vi "NIMS_NS_fir_minphase.vi"(5 "Function name":string, 6 "Line number":i32, 7 "Number of outputs requested":i32, 8 "error in (no error)":errorcluster, 11 "[A]":variant[](array[variant])) -> (0 "error out":errorcluster, 3 "[funct(A)]":variant[](array[variant]))   [LabVIEW 2017]
uses:
  <vilib>/imath/engines/lvmath/Functions/Error Handling/error.ctl
  <instcachedir>/0/NIMS_RunTimeType_From StrictType (excl LVString)_1019F277F0A747EDBCA0F6C52CA54500.lvgen/NIMS_RunTimeType_From StrictType (excl LVString)_1019F277F0A747EDBCA0F6C52CA54500_000.vi
  <instcachedir>/0/NIMS_Get Any Vector_w Error - Matrix_9FDB8FBE264C42EDBC8FF9BA66C3EF33.lvgen/NIMS_Get Any Vector_w Error - Matrix_9FDB8FBE264C42EDBC8FF9BA66C3EF33_001.vi
  <instcachedir>/0/NIMS_Complex To Real_BE01396FDE034E8E94CEBBA1E368668D.lvgen/NIMS_Complex To Real_BE01396FDE034E8E94CEBBA1E368668D_000.vi
  <instcachedir>/0/NIMS_RunTimeType_To Numeric_1CBDAFC4EFAD4045A1DE52278D16738D.lvgen/NIMS_RunTimeType_To Numeric_1CBDAFC4EFAD4045A1DE52278D16738D_000.vi
  <vilib>/addons/Digital Filter Design/NI_DigFilter_MathScript.lvlib
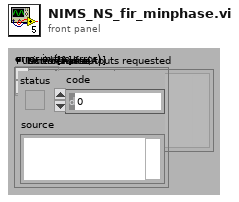
[diagram p1: front panel]
types:
  T1 = typedef "error.ctl" = enum16{"No Error", "Problem", "Input type must not be void", "Incorrect number of parameters", "Function not defined for non-numeric types", "An output variable of the user-defined function is undefined", "Function only defined for character arrays", "Function not defined for boolean, character, or single precision", "Function not defined for complex types", "Not a valid operation", "Inputs must be scalar", "Input matrices are not the same size", "Function only available on RT", "Input matrices must be nonnegative integers of the same type", "Arguments must be non-negative integers less than bitmax", "Number to complement must be less than 2^N", "Bit to get is outside range", "Bit to set is outside range", "Input must be real type ", "At least one parameter must be scalar", "Unable to display plug-in data on RT", "Function not defined for higher dimensional matrices", "Invalid attributes", "Wrong Type of Input Arguments", "Wrong Argument Option", "Invalid file identifier", "Indices must be real positive integers", "The variable is not a matrix data type.", "Number of elements must be the same for indices and values", "You cannot replace elements of a matrix with non-matrix data types.", "Cannot resize a 2D matrix with a linear index", "Unknown variable or symbol", "Indices out of range", "Empty matrix deletion can not be used with two indices", "Number of rows and columns must be the same for indices and values.", "Complex cannot be converted to Boolean", "Char cannot be converted to Boolean", "int64 cannot be converted to Boolean", "uint64 cannot be converted to Boolean", "You cannot convert a Boolean to a character.", "Incompatible input size in 3D surface function", "All rows must have the same number of columns", "Incompatible types", "Invalid matrix dimensions", "Dimension must be 1 or 2", "Base must be an integer between 2 and 36", "Invalid input", "Square matrix required", "Function 'timerstart' must be called before 'timerstop'", "Arguments must be positive real", "Step must not be zero", "Wrong number of input arguments", "Wrong number of output arguments", "Too many index arguments", "Input scalar must be >= 0", "Input scalar must be positive", "Input scalar must not be 0", "Input scalar must be in range [0,1]", "Can't use conditionally defined variable that's undefined", "Input must be a vector", "RT Exec Trace Toolkit not licensed", "Empty vector error", "All elements must be in domain [-1,1]", "All real elements of input vector must be >= 0", "All elements of input vector must be positive", "Values of input vectors are not compatible", "DAQmx not installed", "Input vector must be an increasing vector", "Dereferenced field does not exist within the struct", "A vector or matrix of structures must be indexed before it can be dereferenced", "Lenths of two input vectors are not compatible", "Invalid fieldname", "Empty matrix error", "Cannot use '.' on a type other than Struct", "Unused074", "Data type of the struct's field name is invalid", "Using . to dereference data that is not a struct", "Input struct contains invalid type ", "Size of input matrix is incompatible with input size", "Invalid format specifier", "Could not find field within struct", "Bad permutation array", "Mismatched fieldnames", "ode: User Function could not be opened", "ode: User Function signature does not meet ode requirements", "Unused085", "RunTime: MathScript could not be compiled", "Unknown function", "Only scalars and strings supported", "ode: User Function signature has incorrect number of inputs", "ode:User Function signature has incorrect number of outputs", "Range is too large", "End used without variable", "Function not available (RTE)", "Custom user error", "Arguments must be integers less than bitmax", "Shared library not found", "Header file not found", "Shared library already loaded", "Shared library not loaded", "Shared library function not found", "Shared library string return problem", "Problem calling shared library function", "Problem loading shared library from OS", "Problem parsing shared library header file", "Shared library incompatible types", "Shared library unsupported return type", "Shared library function not exported", "Shared library unsupported input type", "Problem unloading shared library from OS", "Function only available from UI", "Function specified in argument is missing", "An internal error has occurred", "Invalid object", "Invalid property", "Read-only property", "A break command has occurred", "A continue command has occurred", "A return command has occurred", "ode: times parameter invalid", "Function specified in argument has incorrect signature", "Function not found in file", "Reserved keyword cannot be defined as variable", "Reserved keyword cannot be defined as a function or script", "Arguments must be string literals", "Function not supported on this platform", "All columns must have the same number of rows", "Function ignored in RTE warning", "Cannot use : as a parameter that is not a variable", "Output can't be coerced to requested type", "Function not supported on current target", "Variable dependent on an unwired function input", "Unused132", "Unused133", "Unused134", "Unused135", "Unused136", "Unused137", "Unused138", "Unused139", "Global/Persistent must only take constants as arguments.", "Varargin must be last input in the function definition.", "Varargout must be last output in the function definition.", "Invalid output type. Cannot output a cell array of any type other than string.", "Invalid output type. Type is a dynamic struct.", "Invalid output type. Type is a struct that has a field whose type is not known until run-time", "Invalid output type. Type is a struct that has a field which is a plot object.", "MathScript parser DLL missing", "MathScript requires LabVIEW Full", "MathScript license is invalid or missing", "Varargout not supported except in assignments."}
  T2 = typedef "NIMS_CH_character datatype.ctl" = cluster{"Numeric":u8}
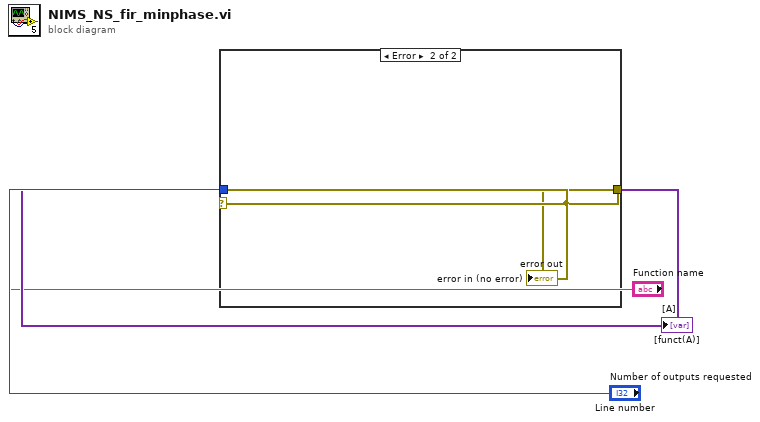
[diagram p0: block diagram]
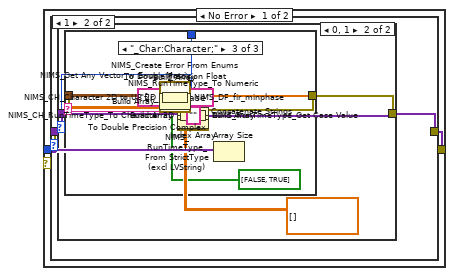
[diagram p2: hidden frame]
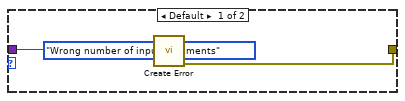
[diagram p3: hidden frame]
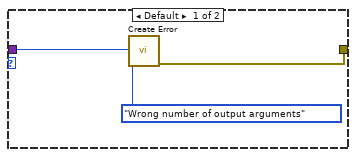
[diagram p4: hidden frame]
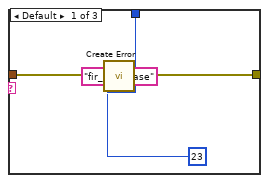
[diagram p5: hidden frame]
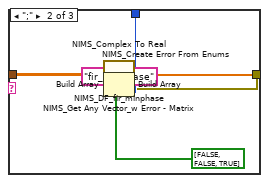
[diagram p6: hidden frame]
diagram:
  n1 = case shown="Error" "error in (no error)" {
    selector: "error in (no error)" -> [_ w84]
    tunnel: [w15 _] -> w4
    tunnel: [w14 w84] -> w3
    tunnel: "error in (no error)" -> [w13 _]
    tunnel: "Number of outputs requested" -> [w12 _]
    tunnel: "[A]" -> [w11 _]
    tunnel: "Function name" -> [w10 _]
    tunnel: "Line number" -> [w9 _]
    frame No Error {
      n2 = Array Size(array=w11) -> (size(s)=w8:i32)
      n3 = case shown="1" w8 {
        tunnel: [_ w27] -> w15
        tunnel: w10 -> [w19 w24]
        tunnel: w9 -> [w20 w25]
        tunnel: w13 -> [w17 w23]
        tunnel: [w16 w22] -> w14
        tunnel: w12 -> [_ w21]
        tunnel: w11 -> [_ w26]
        frame Default {
          n4 = call <vilib>:"Create Error.vi"("Function name"=w19, "error in (no error)"=w17, "Error Enum"=error."Wrong number of input arguments", "Line number"=w20) -> ("error out"=w16:errorcluster)  [unwired: 6 in, 1 out]
        }
        frame 1 {
          n5 = case shown="0, 1" w21 {
            tunnel: [_ w33] -> w27
            tunnel: w24 -> [w31 _]
            tunnel: w25 -> [w32 w47]
            tunnel: w23 -> [w29 w45]
            tunnel: [w28 w39] -> w22
            tunnel: w26 -> [_ w48]
            frame Default {
              n6 = call <vilib>:"Create Error.vi"("Function name"=w31, "error in (no error)"=w29, "Error Enum"=error."Wrong number of output arguments", "Line number"=w32) -> ("error out"=w28:errorcluster)  [unwired: 6 in, 1 out]
            }
            frame 0, 1 {
              n7 = Index Array(array=w48) -> (element=w44:variant)  [unwired: 1 in]
              n8 = call <vilib>:"NIMS_RunTimeType_Get Case Value.vi"("Data In"=w44) -> ("Case Value"=w40:string)  [unwired: 9 in, 1 out]
              n9 = call <vilib>:"NIMS_CH_RunTimeType_To Character 2D.vi"("Variant"=w44) -> ("data"=w41:T2[][])  [unwired: 1 in]
              n10 = call-generic <vilib>:"NIMS_RunTimeType_To Numeric.vi"("DataType"=cdb[][] [], "Variant"=w44) -> ("data"=w42:cdb[][])  [unwired: 1 in]
              n11 = Concatenate Strings(w40) -> (w46:string)
              n12 = case shown="\"_Char:Character;\"" w46 {
                tunnel: w45 -> [w50 w59 w74]
                tunnel: [_ w54 w69] -> w38
                tunnel: [w49 w55 w70] -> w39
                tunnel: w42 -> [_ w67 _]
                tunnel: w41 -> [_ _ w82]
                tunnel: w47 -> [w53 w62 w77]
                frame Default {
                  n13 = call <vilib>:"Create Error.vi"("Function name"="fir_minphase", "error in (no error)"=w50, "Error Enum"=23, "Line number"=w53) -> ("error out"=w49:errorcluster)  [unwired: 6 in, 1 out]
                }
                frame ";" {
                  w57 = "fir_minphase"
                  n14 = call-generic <vilib>:"NIMS_Complex To Real.vi"("A"=w67) -> ("Error Enum"=w65:T1, "Real(A)"=w66:dbl[][])  [unwired: 8 in, 1 out]
                  n15 = call-generic <vilib>:"NIMS_Get Any Vector_w Error - Matrix.vi"("A"=w66) -> ("Error Enum"=w64:T1, "Vector"=w68:dbl[])  [unwired: 8 in, 1 out]
                  n16 = call <vilib>:"NIMS_DF_fir_minphase.vi"("b1"=w68) -> ("error"=w63:i32, "b2"=w54:dbl[])  [unwired: 9 in]
                  n17 = Build Array(w57, w57, "fir_minphase") -> (w60:string[])
                  n18 = Build Array(w65, w64, w63) -> (w61:i32[])
                  n19 = call <vilib>:"NIMS_Create Error From Enums.vi"("Error Code"=bool[] [FALSE, FALSE, TRUE], "error in (no error)"=w59, "Line no"=w62, "Error Enums"=w61, "Function names"=w60) -> ("error out"=w55:errorcluster)  [unwired: 6 in]
                }
                frame "_Char:Character;" {
                  n20 = call <vilib>:"NIMS_CH_Character 2D to U8 2D.vi"("Character 2D array"=w82) -> ("U8 2D array"=w81:u8[][])  [unwired: 10 in]
                  n21 = To Double Precision Float(number=w81) -> (double precision float=w80:dbl[][])
                  n22 = call-generic <vilib>:"NIMS_Get Any Vector_w Error - Matrix.vi"("A"=w80) -> ("Error Enum"=w79:T1, "Vector"=w83:dbl[])  [unwired: 8 in, 1 out]
                  n23 = call <vilib>:"NIMS_DF_fir_minphase.vi"("b1"=w83) -> ("error"=w78:i32, "b2"=w69:dbl[])  [unwired: 9 in]
                  n24 = Build Array("fir_minphase", "fir_minphase") -> (w75:string[])
                  n25 = Build Array(w79, w78) -> (w76:i32[])
                  n26 = call <vilib>:"NIMS_Create Error From Enums.vi"("Error Code"=bool[] [FALSE, TRUE], "error in (no error)"=w74, "Line no"=w77, "Error Enums"=w76, "Function names"=w75) -> ("error out"=w70:errorcluster)  [unwired: 6 in]
                }
              }
              n27 = Build Array(w38) -> (w37:dbl[][])
              n28 = To Double Precision Complex(1:w37) -> (0:w36:cdb[][])
              n29 = call-generic <vilib>:"NIMS_RunTimeType_From StrictType (excl LVString).vi"("Plug-In Name"="", "Data In"=w36) -> ("Data Out"=w34:variant)  [unwired: 2 in]
              n30 = Build Array(w34) -> (w33:variant[])
            }
          }
        }
      }
    }
    frame Error {
    }
  }
  "error out" <- w3
  "[funct(A)]" <- w4
